vi "XL320_Read Word From 2 Addresses.vi"(8 "Error in (no error)":errorcluster, 9 "Address number (0)":u16, 10 "Motor ID (0)":u8, 11 "VISA resource name":refnum<visa-resource-name>) -> (0 "error out":errorcluster, 2 "Data":u16, 3 "VISA resource name out":refnum<visa-resource-name>)   [LabVIEW 2017, in "Dynamixel XL320.lvlib"]
doc: "Reads a word type (U16) from two addresses of a Dynamixel motor. The value returned will typically range from 0 to 1023. This VI assumes little endian byte order. This is a Low-Level VI that is used by other VIs."
uses:
  <instrlib>/Dynamixel XL320 (Drivers instrument)/Dynamixel XL320.lvlib
panel:
  # "Ghislain REMY, IUT de Cachan, 2015 December 2015"
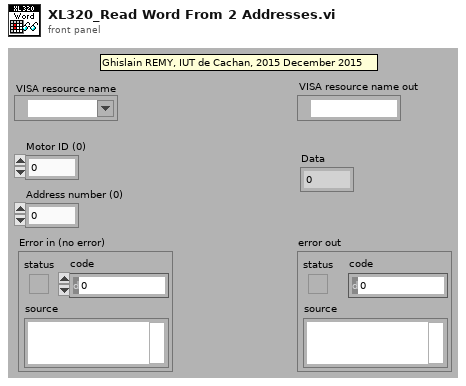
[diagram p1: front panel]
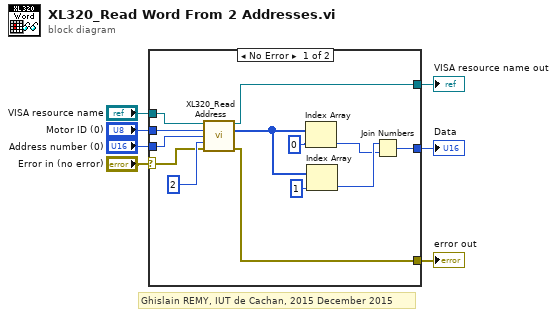
[diagram p0: block diagram]
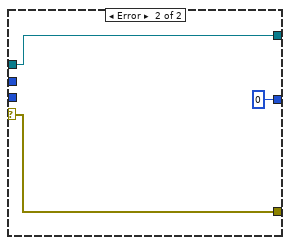
[diagram p2: hidden frame]
diagram:
  # "Ghislain REMY, IUT de Cachan, 2015 December 2015"
  n1 = case shown="No Error" "Error in (no error)" {
    selector: "Error in (no error)" -> [w8 w23]
    tunnel: [w16 u16 0] -> w7
    tunnel: "VISA resource name" -> [w12 w22]
    tunnel: [w15 w22] -> w5
    tunnel: [w13 w23] -> w4
    tunnel: "Address number (0)" -> [w10 _]
    tunnel: "Motor ID (0)" -> [w11 _]
    frame No Error {
      n2 = call <instrlib>:"XL320_Read Address.vi"("VISA resource name"=w12, "Motor ID (0)"=w11, "Address number (0)"=w10, "Number of Addresses to read (1)"=u16 2, "Error in (no error)"=w8) -> ("VISA resource name Out"=w15:refnum<visa-resource-name>, "Data Read"=w14:u8[], "error out"=w13:errorcluster)  [unwired: 7 in, 1 out]
      n3 = Index Array(array=w14, index=0) -> (element=w17:u8)
      n4 = Index Array(array=w14, index=1) -> (element=w18:u8)
      n5 = Join Numbers(hi=w18, lo=w17) -> ((hi.lo)=w16:u16)
    }
    frame Error {
    }
  }
  "Data" <- w7
  "VISA resource name out" <- w5
  "error out" <- w4
